vi "Read composition.vi"(5 "Circuit cluster":T1) -> (2 "Composition":string[][](table))   [LabVIEW 2016]
uses:
  TypeDefs/Circuit Cluster.ctl
  Classes/GateAbst/GateAbst.lvclass
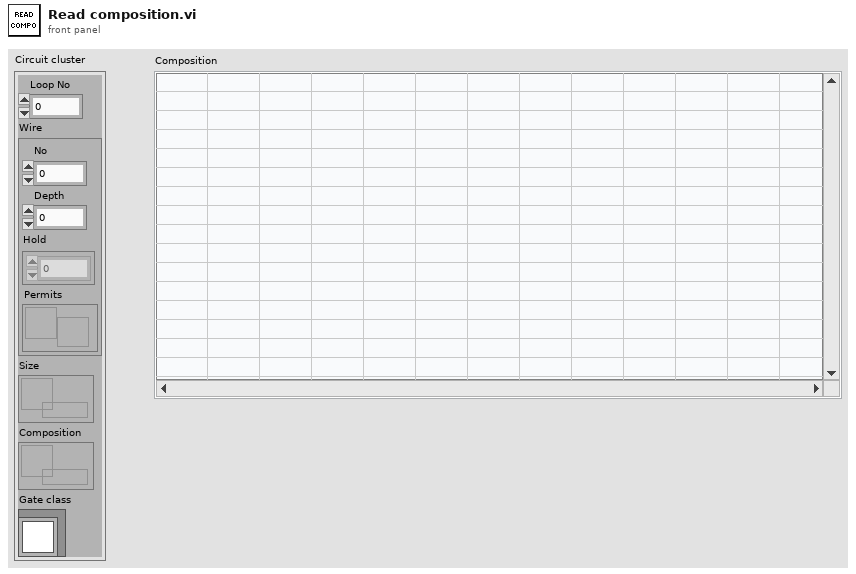
[diagram p1: front panel]
types:
  T1 = typedef "Circuit Cluster.ctl" = cluster{"Loop No":i32, "Wire":cluster{"No":i32, "Depth":i32, "Hold":i32[][], "Permits":refnum<notifier>}, "Size":refnum<queue>, "Composition":refnum<queue>, "Gate class":refnum<class "GateAbst.lvclass">}
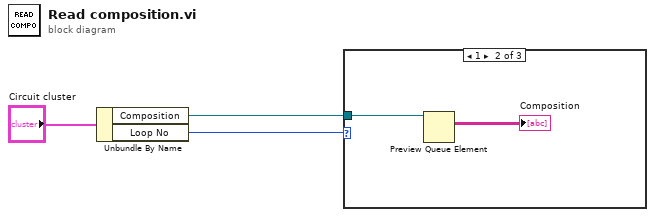
[diagram p0: block diagram]
diagram:
  n1 = Unbundle By Name("Circuit cluster") -> ("Composition"=w2:refnum<queue>, "Loop No"=w1:i32)
  n2 = case shown="1" w1 {
    tunnel: w2 -> [_ w5 _]
    frame 0 {
    }
    frame 1 {
      n3 = Preview Queue Element(queue=w5) -> (element=→"Composition":string[][])  [unwired: 2 in, 3 out]
    }
    frame Default {
    }
  }
